vi "ZiptIt.vi"(9 "Folder to zip":path, 11 "Zip file":path) -> (0 "error out":errorcluster, 3 "Generated Zip File":path)   [LabVIEW 2022 SP3]
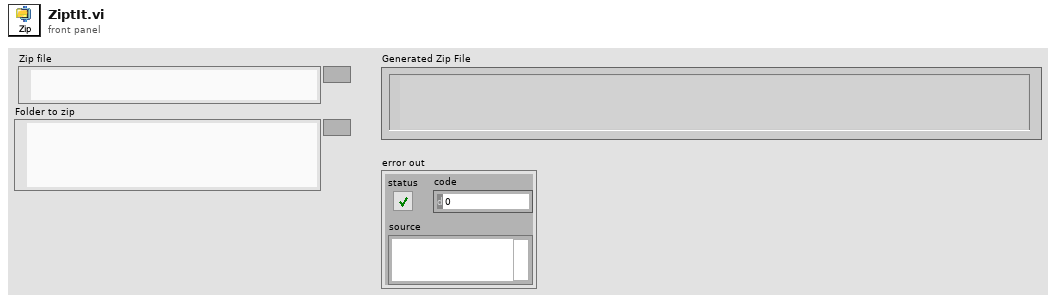
[diagram p1: front panel]
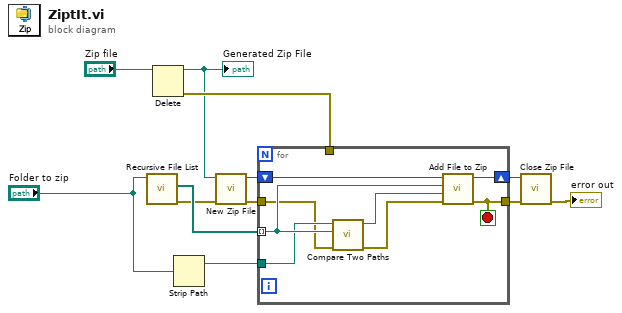
[diagram p0: block diagram]
diagram:
  n1 = call <vilib>:"Recursive File List.vi"("Folder Path"="Folder to zip") -> ("error out"=w6:errorcluster, "All Files in Dir"=w7:path[])  [unwired: 6 in, 3 out]
  n2 = Delete(path (use dialog)="Zip file") -> (deleted path=w9:path, error out=w11:errorcluster)  [unwired: 4 in, 1 out]
  "Generated Zip File" <- w9
  n3 = Strip Path(path="Folder to zip") -> (stripped path=w10:path)  [unwired: 1 out]
  n4 = call <vilib>:"New Zip File.vi"("error in (no error)"=w6, "target"=w9) -> ("error out"=w3:errorcluster, "zip file out"=w2:i64)  [unwired: 1 in, 3 out]
  n5 = for {
    tunnel: w7 -> [w17] mode=indexing
    tunnel: w3 -> [w14]
    tunnel: [w18] -> w4
    shift-right: [w19] -> w5
    shift-left: w2 -> [w20]
    tunnel: w10 -> [w16]
    tunnel: w11 -> [_]
    stop <- w18 stop-if-true
    n6 = call <vilib>:"Compare Two Paths.vi"("error in (no error)"=w14, "Path 2"=w17, "Path 1"=w16) -> ("error out"=w13:errorcluster, "Relative Path from 1 to 2"=w15:path)  [unwired: 5 in, 2 out]
    n7 = call <vilib>:"Add File to Zip.vi"("error in (no error)"=w13, "destination path in zip"=w15, "source file path"=w17, "zip file in"=w20) -> ("error out"=w18:errorcluster, "zip file out"=w19:i64)  [unwired: 6 out]
  }
  n8 = call <vilib>:"Close Zip File.vi"("error in (no error)"=w4, "zip file in"=w5) -> ("error out"=→"error out":errorcluster)  [unwired: 1 in, 4 out]
